vi "Excel_Create_Workbook.vi"(8 "error in (no error)":errorcluster, 10 "Path":path, 11 "excel application":refnum<k7>) -> (0 "error out":errorcluster, 3 "references":T1)   [LabVIEW 2010, in "NI_ReportGenerationToolkit.lvlib"]
uses:
  <vilib>/addons/_office/NI_ReportGenerationToolkit.lvlib
panel:
  in  "Excel._Worksheet":refnum<k7>
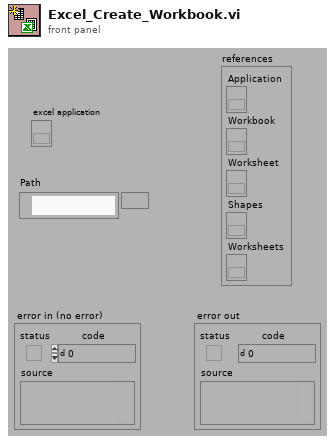
[diagram p1: front panel]
types:
  T1 = cluster{"Application":refnum<k7>, "Workbook":refnum<k7>, "Worksheet":refnum<k7>, "Shapes":refnum<k7>, "Worksheets":refnum<k7>}
  T2 = cluster{"excel application":refnum<k7>, "Add":refnum<k7>, "Excel._Worksheet":refnum<k7>, "Shapes":refnum<k7>, "Worksheets":refnum<k7>}
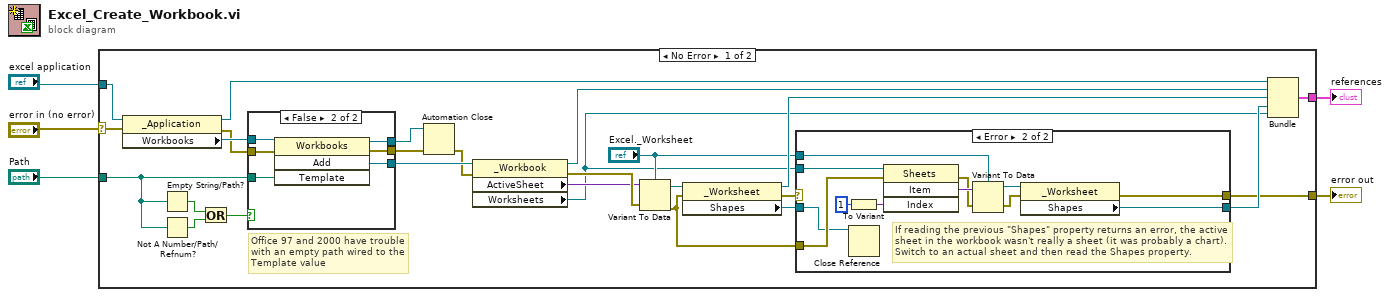
[diagram p0: block diagram]
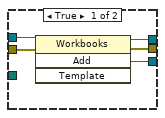
[diagram p2: hidden frame]
diagram:
  n1 = case shown="No Error" "error in (no error)" {
    selector: "error in (no error)" -> [w10 w57]
    tunnel: "excel application" -> [w27 _]
    tunnel: "Path" -> [w9 _]
    tunnel: [w18 _] -> w3
    tunnel: [w13 w57] -> w2
    frame No Error {
      # "Office 97 and 2000 have trouble\nwith an empty path wired to the\nTemplate value"
      n2 = property class="_Application"(reference=w27, error in=w10) -> (reference out=w28:refnum<k7>, error out=w29:errorcluster, "Workbooks"=w30:refnum<k7>)
      n3 = Empty String/Path?(string/path=w9) -> (empty?=w8:bool)
      n4 = Not A Number/Path/Refnum?(number/path/refnum=w9) -> (NaN/Path/Refnum?=w7:bool)
      n5 = Or(x=w8, y=w7) -> (x .or. y?=w6:bool)
      n6 = case shown="False" w6 {
        tunnel: [w36 w42] -> w31
        tunnel: w30 -> [w35 w41]
        tunnel: w29 -> [w34 w40]
        tunnel: [w33 w39] -> w26
        tunnel: [w32 w38] -> w25
        tunnel: w9 -> [_ w37]
        frame True {
          n7 = invoke class="Workbooks" method="Add"(reference=w35, error in=w34) -> (reference out=w32:refnum<k7>, error out=w33:errorcluster, "Add"=w36:refnum<k7>)  [unwired: 2 in, 1 out]
        }
        frame False {
          n8 = invoke class="Workbooks" method="Add"(reference=w41, error in=w40, "Template"=w37) -> (reference out=w38:refnum<k7>, error out=w39:errorcluster, "Add"=w42:refnum<k7>)  [unwired: 1 in, 1 out]
        }
      }
      n9 = Automation Close(3:w26, 5:w25) -> (0:w24:errorcluster)
      n10 = property class="_Workbook"(reference=w31, error in=w24) -> (reference out=w20:refnum<k7>, error out=w23:errorcluster, "ActiveSheet"=w21:variant, "Worksheets"=w11:refnum<k7>)
      n11 = Variant To Data(error in=w23, Variant=w21, type="Excel._Worksheet") -> (error out=w17:errorcluster, data=w22:refnum<k7>)
      n12 = property class="_Worksheet"(reference=w22, error in=w17) -> (reference out=w19:refnum<k7>, error out=w14:errorcluster, "Shapes"=w16:refnum<k7>)
      n13 = case shown="Error" w14 {
        selector: w14 -> [w44 _]
        tunnel: w11 -> [_ w53]
        tunnel: "Excel._Worksheet" -> [_ w51]
        tunnel: [w43 w50] -> w15
        tunnel: [w44 w49] -> w13
        tunnel: w17 -> [_ w48]
        tunnel: w16 -> [w43 w47]
        frame No Error {
        }
        frame Error {
          # "If reading the previous \"Shapes\" property returns an error, the active\nsheet in the workbook wasn't really a sheet (it was probably a chart).\nSwitch to an actual sheet and then read the Shapes property."
          n14 = To Variant(anything=1) -> (Variant=w55:variant)
          n15 = Close Reference(reference=w47) -> ()  [unwired: 1 in, 1 out]
          n16 = invoke class="Sheets" method="Item"(reference=w53, error in=w48, "Index"=w55) -> (error out=w52:errorcluster, "Item"=w56:variant)  [unwired: 1 in, 2 out]
          n17 = Variant To Data(error in=w52, Variant=w56, type=w51) -> (error out=w45:errorcluster, data=w46:refnum<k7>)
          n18 = property class="_Worksheet"(reference=w46, error in=w45) -> (error out=w49:errorcluster, "Shapes"=w50:refnum<k7>)  [unwired: 1 out]
        }
      }
      n19 = Bundle("excel application"=w28, "Add"=w20, "Excel._Worksheet"=w19, "Shapes"=w15, "Worksheets"=w11) -> (w18:T2)  [unwired: 1 out]
    }
    frame Error {
    }
  }
  "error out" <- w2
  "references" <- w3
